vi "Deploy SV Libraries.vi"(8 "error in (no error)":errorcluster, 11 "SV B-M in":refnum<class "SV B-M (Host).lvclass">) -> (0 "error out":errorcluster, 3 "SV B-M out":refnum<class "SV B-M (Host).lvclass">)   [LabVIEW 2015, in "SV B-M (Host).lvclass"]
doc: "Deploy SV libraries to either the target or host depending on sequence parameter specification."
uses:
  SV B-M (Host).lvclass
  SV B-M (Host).lvclass/SV B-M (Host).ctl
  Listbox - In Progress.vi
  Listbox - Complete.vi
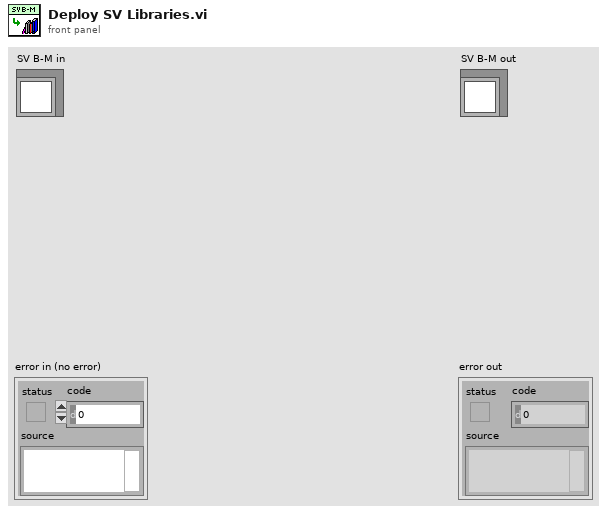
[diagram p1: front panel]
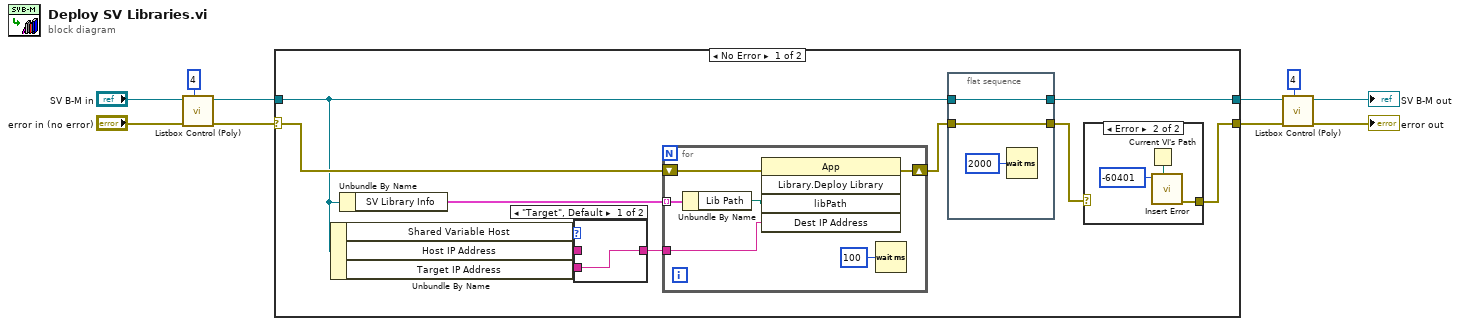
[diagram p0: block diagram]
diagram:
  n1 = call-poly "Listbox Control (Poly).vi"("Row to Update"=4, "error in (no error)"="error in (no error)", "SV B-M In"="SV B-M in") -> ("error out"=w7:errorcluster, "SV B-M Out"=w9:refnum<class "SV B-M (Host).lvclass">)  [unwired: 7 in]
  n2 = case shown="No Error" w7 {
    selector: w7 -> [w16 w37]
    tunnel: [w15 w38] -> w4
    tunnel: w9 -> [w14 w38]
    tunnel: [w11 w37] -> w2
    frame No Error {
      n3 = Unbundle By Name(w14) -> ("Shared Variable Host"=w21:enum16{"Target", "Host"}, "Host IP Address"=w20:string, "Target IP Address"=w19:string)
      n4 = Unbundle By Name(w14) -> ("SV Library Info"=w18:cluster{"Lib Path":path, "Lib Size":u16}[])
      n5 = case shown="\"Target\", Default" w21 {
        tunnel: w20 -> [_ w36]
        tunnel: w19 -> [w35 _]
        tunnel: [w35 w36] -> w17
        frame "Target", Default {
        }
        frame "Host" {
        }
      }
      n6 = for {
        tunnel: w18 -> [w34] mode=indexing
        tunnel: w17 -> [w30]
        shift-right: [w32] -> w13
        shift-left: w16 -> [w33]
        n7 = Unbundle By Name(w34) -> ("Lib Path"=w31:path)
        n8 = invoke class="App" method="Library.Deploy Library"(error in=w33, "libPath"=w31, "Dest IP Address"=w30) -> (error out=w32:errorcluster)  [unwired: 2 in, 4 out]
        n9 = Wait (ms)(milliseconds to wait=u32 100) -> ()  [unwired: 1 out]
      }
      n10 = flat-sequence {
        tunnel: [w27] -> w12
        tunnel: w13 -> [w27]
        tunnel: [w26] -> w15
        tunnel: w14 -> [w26]
        frame #0 {
          n11 = Wait (ms)(milliseconds to wait=u32 2000) -> ()  [unwired: 1 out]
        }
      }
      n12 = case shown="Error" w12 {
        selector: w12 -> [w22 _]
        tunnel: [w22 w24] -> w11
        frame No Error {
        }
        frame Error {
          n13 = Current VI's Path() -> (path=w23:path)
          n14 = call "Insert Error.vi"("VI Path"=w23, "Error Code"=-60401) -> ("error out"=w24:errorcluster)  [unwired: 9 in]
        }
      }
    }
    frame Error {
    }
  }
  n15 = call-poly "Listbox Control (Poly).vi"("Row to Update"=4, "error in (no error)"=w2, "SV B-M In"=w4) -> ("error out"=→"error out":errorcluster, "SV B-M Out"=→"SV B-M out":refnum<class "SV B-M (Host).lvclass">)  [unwired: 7 in]
